vi "analog-read-1-chan.vi"(7 "Analog Ref Override (V)":dbl, 8 "Error In":errorcluster, 10 "Analog Channel":u8, 11 "LINX Resource":T1) -> (0 "Error Out":errorcluster, 1 "AI Ref":dbl, 2 "Voltage":dbl, 3 "LINX Resource":T1)   [LabVIEW 2014, in "LMH-LINX.lvlib"]
doc: "Read the value of the specified analog input channel."
uses:
  <vilib>/MakerHub/LINX/LMH-LINX.lvlib
  <vilib>/MakerHub/LINX/Private/Type Defs/LINX Ref.ctl
  <vilib>/MakerHub/LINX/Private/Type Defs/Platform.ctl
  <vilib>/MakerHub/LINX/Private/Type Defs/Interface.ctl
  <vilib>/MakerHub/LINX/Private/Device/Type Defs/LINX Device Config.ctl
  <vilib>/MakerHub/LINX/Private/Device/Type Defs/TCP Config.ctl
  <vilib>/MakerHub/LINX/Private/Device/Type Defs/Channels.ctl
  <vilib>/MakerHub/LINX/Private/Local IO/LinxAnalogRead.vi
  <vilib>/MakerHub/LINX/Public/Utilities/Check Channel.vi
  <vilib>/MakerHub/LINX/Private/Device/Peripheral/Analog/Analog Read.vi
  <vilib>/MakerHub/LINX/Private/Utilties/Generate Error.vi
  <vilib>/MakerHub/LINX/Private/Device/Device.lvlib
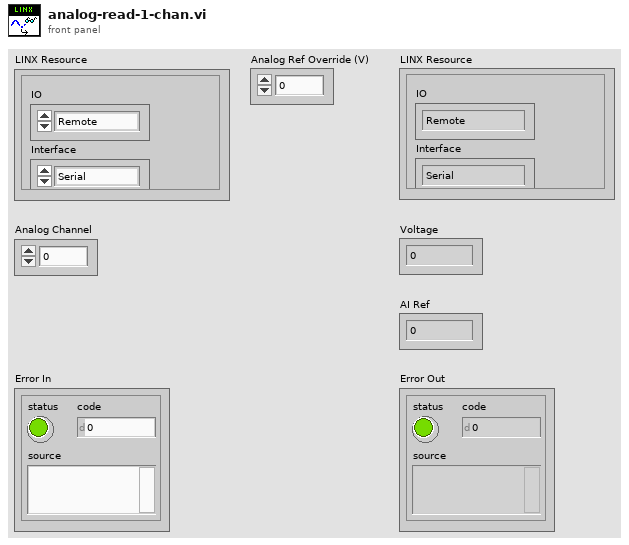
[diagram p1: front panel]
types:
  T1 = typedef "LMH-LINX.lvlib/LINX Ref.ctl" = cluster{"IO":T2, "Interface":T3, "LINX Device Config":T4}
  T2 = typedef "LMH-LINX.lvlib/Platform.ctl" = enum16{"Remote", "Local"}
  T3 = typedef "LMH-LINX.lvlib/Interface.ctl" = enum16{"Serial", "TCP"}
  T4 = typedef "LMH-LINX.lvlib/Device.lvlib/LINX Device Config.ctl" = cluster{"Interface":T3, "COM Port":refnum<visa-resource-name>, "TCP Configuration":T5, "Device Family":u8, "Device ID":u8, "Device Name":string, "TCP Ref":refnum<k5>, "Channels":T6}
  T5 = typedef "LMH-LINX.lvlib/Device.lvlib/TCP Config.ctl" = cluster{"IP Address":string, "Port":u16}
  T6 = typedef "LMH-LINX.lvlib/Channels.ctl" = cluster{"DI":u8[], "DO":u8[], "AI":u8[], "AO":u8[], "PWM":u8[], "QE":u8[], "UART":u8[], "I2C 2":u8[], "SPI":u8[], "CAN":u8[], "Servo":u8[], "AI Ref (V)":dbl, "AI Resolution (Bits)":u8, "AO Ref (V)":dbl, "AO Resolution (Bits)":u8}
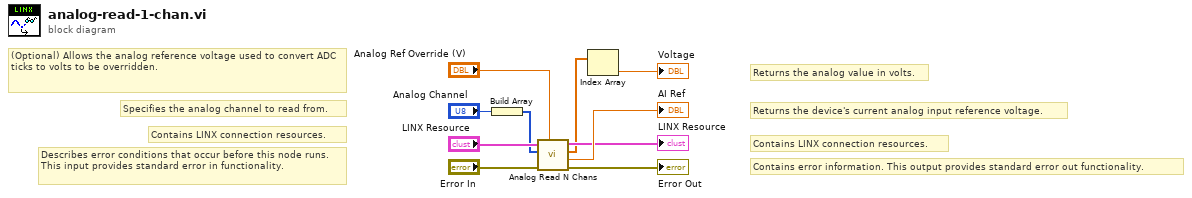
[diagram p0: block diagram]
diagram:
  # "(Optional) Allows the analog reference voltage used to convert ADC ticks to volts to be overridden."
  # "Specifies the analog channel to read from."
  # "Returns the analog value in volts."
  # "Returns the device's current analog input reference voltage."
  # "Contains LINX connection resources."
  # "Contains error information. This output provides standard error out functionality."
  # "Contains LINX connection resources."
  # "Describes error conditions that occur before this node runs. This input provides standard error in functionality."
  n1 = Build Array("Analog Channel") -> (w3:u8[])
  n2 = call <vilib>:"Analog Read N Chans.vi"("Analog Ref Override"="Analog Ref Override (V)", "Error In"="Error In", "AI Channel(s)"=w3, "LINX Resource"="LINX Resource") -> ("Error Out"=→"Error Out":errorcluster, "AI Ref"=→"AI Ref":dbl, "Voltages"=w2:dbl[], "LINX Resource"=→"LINX Resource":T1)  [unwired: 4 in]
  n3 = Index Array(array=w2) -> (element=→"Voltage":dbl)  [unwired: 1 in]
